vi "Constants.vi"() -> ()   [LabVIEW 2015, in "DMM-SWITCH-ScanList Shared.lvlib"]
doc: "Use this Global VI to access the GUIDs assigned to the page resources of the Custom Device."
uses:
  DMM-SWITCH-ScanList Shared.lvlib
  <instrlib>/niDMM/nidmm.llb/niDMM Function.ctl
  <instrlib>/niDMM/nidmm.llb/niDMM Resolution in Digits.ctl
  <instrlib>/niSwitch/niSwitch.LLB/niSwitch Topologies.ctl
  <instrlib>/niSwitch/niSwitch.LLB/niSwitch Trigger Input.ctl
  <instrlib>/niSwitch/niSwitch.LLB/niSwitch Scan Advanced Output.ctl
  <instrlib>/niDMM/nidmm.llb/niDMM Measurement Complete.ctl
  <instrlib>/niDMM/nidmm.llb/niDMM Trigger.ctl
panel:
  in  "Tab Control":T1(tab)
  in  "GUID Runtime Iteration":string="5260A2FF-FA1A-4B8D-AACD-153CF615834C"
  in  "GUID Runtime Error Status":string="5260A2FF-FA1A-4B8D-AACD-153CF615834C"
  in  "GUID Runtime Error Code":string="5260A2FF-FA1A-4B8D-AACD-153CF615834C"
  in  "GUID Initialization Error Status":string="5260A2FF-FA1A-4B8D-AACD-153CF615834C"
  in  "GUID Initialization Error Code":string="5260A2FF-FA1A-4B8D-AACD-153CF615834C"
  in  "GUID Scan Trigger":string="5260A2FF-FA1A-4B8D-AACD-153CF615834C"
  in  "GUID Group Ch - Runtime Status":string="813CC596-1D51-426F-B292-57396C68DA7F"
  in  "GUID Group Ch - Measurement Channels":string="3C436B89-AF05-4727-AB74-6F367A82FA29"
  in  "GUID Group Ch - Input Channels":string="247BA5C3-EBA8-4DAA-B4FA-14FAA185E47F"
  in  "GUID Group Ch - Configuration":string="5260A2FF-FA1A-4B8D-AACD-153CF615834C"
  in  "GUID Triggers Configuration Channel":string="5260A2FF-FA1A-4B8D-AACD-153CF615834C"
  in  "GUID Switch Configuration Channel":string="2CD8A1A5-3D89-4F04-ABA6-DE3C84A9E458"
  in  "GUID DMM Configuration Channel":string="F70F49EF-EA01-4EE0-9516-062BB723C6FA"
  in  "GUID DMM-SWITCH-ScanList":string="b44fa48e-2c45-4166-a547-1c211cfe843f"
  in  "Top Files Relative Path Location":string="National Instruments\\NI-DAQ\\Switch\\TopFiles"
  in  "Output Measurements Channels Path":string="Targets/Controller/Custom Devices/DMM-SWITCH-ScanList/Measurement Channels"
  in  "DMM Range Index":u16
  in  "TRIG DMM Trigger Source":string="TRIG DMM Trigger Source"
  in  "TRIG DMM Measurement Complete":string="TRIG DMM Measurement Complete"
  in  "TRIG SWITCH Scan Advanced Output":string="TRIG SWITCH Scan Advanced Output"
  in  "TRIG SWITCH Trigger Source":string="TRIG SWITCH Trigger Source"
  in  "SWITCH ListBox Channel Items":string="SWITCH ListBox Channel Items"
  in  "SWITCH ListBox Selectable Channel Items":string="SWITCH ListBox Selectable Channel Items"
  in  "SWITCH ab0":string="SWITCH ab0"
  in  "SWITCH Scan List String Mode":string="SWITCH Scan List String Mode"
  in  "SWITCH Model":string="SWITCH Model"
  in  "SWITCH Scan List":string="SWITCH Scan List"
  in  "SWITCH Generated Scan List":string="SWITCH Generated Scan List"
  in  "SWITCH Manual Scan List":string="SWITCH Manual Scan List"
  in  "SWITCH Topology":string="SWITCH Topology"
  in  "SWITCH Resource Name":string="SWITCH Resource Name"
  in  "DMM Range [EU]":string="DMM Range [EU]"
  in  "DMM Resolution in Digits":string="DMM Resolution in Digits"
  in  "DMM Measurement Type":string="DMM Measurement Type"
  in  "DMM Resource Name":string="DMM Resource Name"
  in  "SWITCH ListBox Channel Items Value":string[](array[string])
  in  "SWITCH ListBox Selectable Channel Items Value":string[](array[string])
  in  "SWITCH ab0 Value":bool
  in  "SWITCH Scan List String Mode Value":bool
  in  "SWITCH Switch Model Value":string="2503"
  in  "SWITCH Scan List Value":string
  in  "SWITCH Generated Scan List Value":string
  in  "SWITCH Manual Scan List Value":string="ab0->com0 & com0->ch0:2;"
  in  "SWITCH Topology Value":T2="2503/2-Wire 24x1 Mux" caption="SWITCH Topology"
  in  "DMM Resource Name Value":string="DMM"
  in  "SWITCH Resource Name Value":string="SWITCH"
  in  "DMM Range [EU] Value":dbl=10000.0
  in  "DMM Resolution in Digits Value":T3=6.5 caption="Resolution in Digits" items=["3 1/2"=3.5, "4 1/2"=4.5, "5 1/2"=5.5, "6 1/2"=6.5, "7 1/2"=7.5]
  in  "DMM Measurement Type Value":T4=enum."2-wire Resistance" caption="DMM Measurement Type"
  in  "TRIG SWITCH Trigger Source Value":T5=enum."TTL1" caption="TRIG Switch Trigger Source"
  in  "TRIG SWITCH Scan Advanced Output Value":T6=enum."TTL2" caption="TRIG Scan Advanced Output"
  in  "TRIG DMM Measurement Complete  Value":T7=enum."TTL 1" caption="TRIG DMM Measurement \nComplete Destination"
  in  "TRIG DMM Trigger Source Value":T8=enum."TTL 2" caption="TRIG DMM Trigger Source"
  in  "Group Ch - Runtime Status":string
  in  "Group Ch - Measurement Channels":string
  in  "Group Ch - Input Channels":string
  in  "Group Ch - Configuration":string
  in  "Runtime Status Ch - Runtime Iteration":string
  in  "Runtime Status Ch - Runtime Error Code":string
  in  "Runtime Status Ch - Runtime Error Status":string
  in  "Runtime Status Ch - Initialization Error Code":string
  in  "Runtime Status Ch - Initialization Error Status":string
  in  "Input Ch - Scan Trigger":string
  in  "Config Ch - Triggers Configuration":string
  in  "Config Ch - Switch Configuration":string
  in  "Config Ch - DMM Configuration":string
  # "DMM"
  # "SWITCH"
  # "TIMING & TRIGGERS"
  # "OUTPUT CHANNELS"
  # "CONFIGURATION"
  # "INPUT CHANNELS"
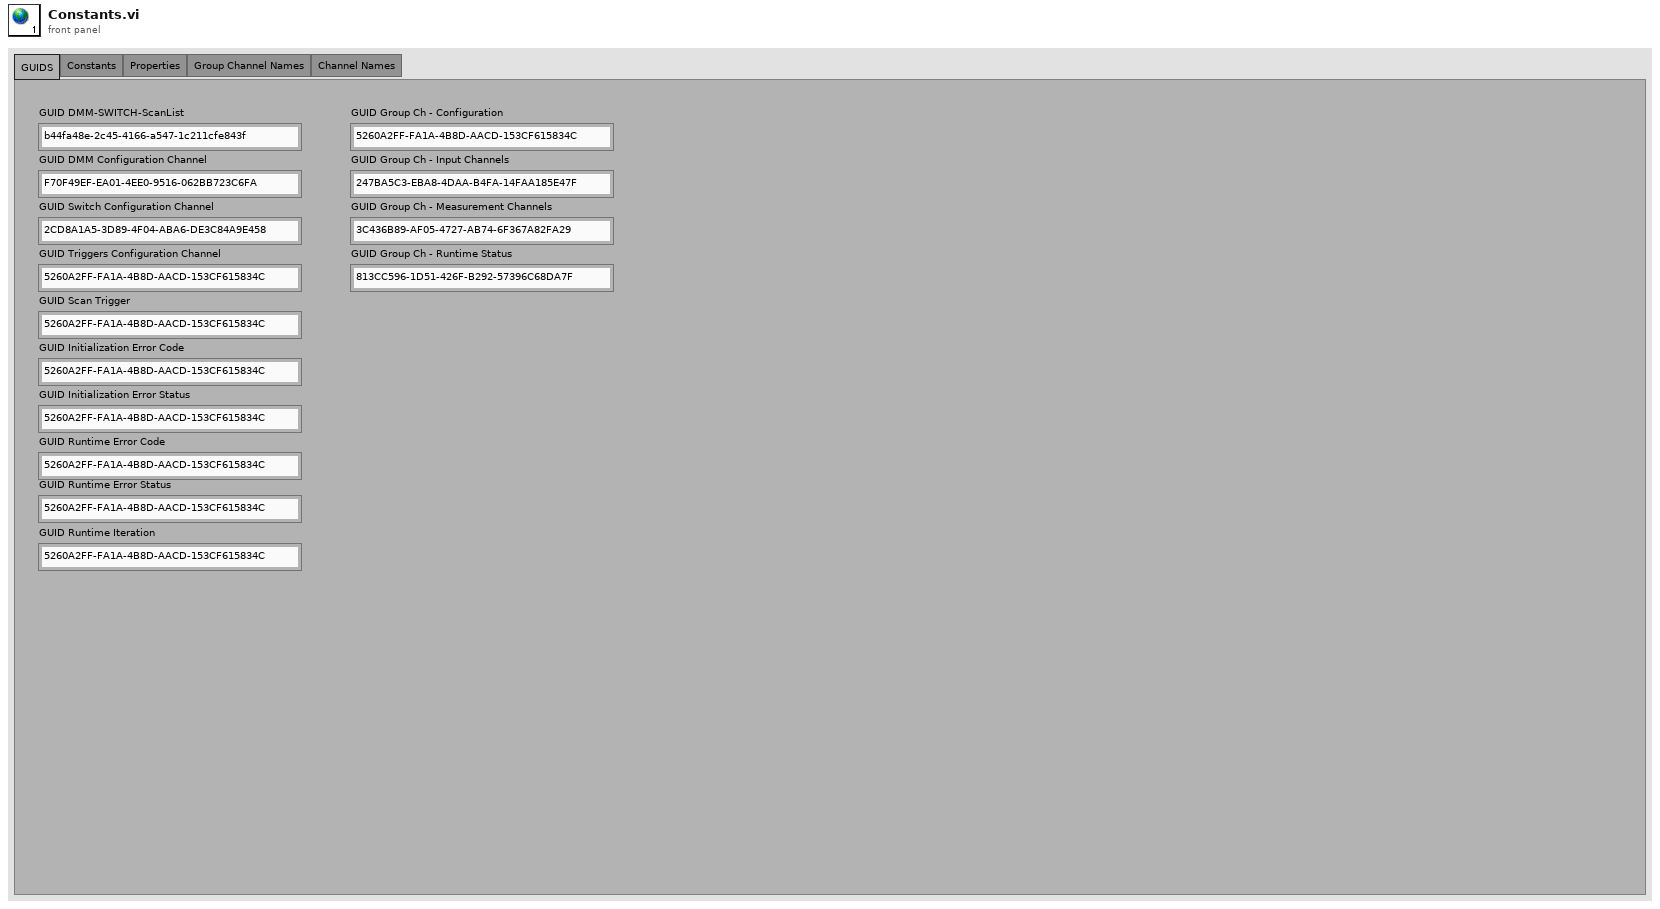
[diagram p1: front panel]
types:
  T1 = enum32{"GUIDS", "Constants", "Properties", "Group Channel Names", "Channel Names"}
  T2 = typedef "niSwitch Topologies.ctl" = string
  T3 = typedef "niDMM Resolution in Digits.ctl" = dbl
  T4 = typedef "niDMM Function.ctl" = enum16{"DC Volts", "AC Volts", "DC Current", "AC Current", "2-wire Resistance", "4-wire Resistance", "Diode", "Frequency", "Period", "AC Volts DC Coupled", "Capacitance", "Inductance", "Temperature"}
  T5 = typedef "niSwitch Trigger Input.ctl" = enum16{"Immediate", "External", "TTL0", "TTL1", "TTL2", "TTL3", "TTL4", "TTL5", "TTL6", "TTL7", "ECL0", "ECL1", "PXI Star", "Software Trigger Function", "Rear Connector", "Front Connector", "Rear Connector of Module 1", "Rear Connector of Module 2", "Rear Connector of Module 3", "Rear Connector of Module 4", "Rear Connector of Module 5", "Rear Connector of Module 6", "Rear Connector of Module 7", "Rear Connector of Module 8", "Rear Connector of Module 9", "Rear Connector of Module 10", "Rear Connector of Module 11", "Rear Connector of Module 12", "Front Connector of Module 1", "Front Connector of Module 2", "Front Connector of Module 3", "Front Connector of Module 4", "Front Connector of Module 5", "Front Connector of Module 6", "Front Connector of Module 7", "Front Connector of Module 8", "Front Connector of Module 9", "Front Connector of Module 10", "Front Connector of Module 11", "Front Connector of Module 12"}
  T6 = typedef "niSwitch Scan Advanced Output.ctl" = enum16{"None", "External", "TTL0", "TTL1", "TTL2", "TTL3", "TTL4", "TTL5", "TTL6", "TTL7", "ECL0", "ECL1", "PXI Star", "Rear Connector", "Front Connector", "Rear Connector Module 1", "Rear Connector Module 2", "Rear Connector Module 3", "Rear Connector Module 4", "Rear Connector Module 5", "Rear Connector Module 6", "Rear Connector Module 7", "Rear Connector Module 8", "Rear Connector Module 9", "Rear Connector Module 10", "Rear Connector Module 11", "Rear Connector Module 12", "Front Connector Module 1", "Front Connector Module 2", "Front Connector Module 3", "Front Connector Module 4", "Front Connector Module 5", "Front Connector Module 6", "Front Connector Module 7", "Front Connector Module 8", "Front Connector Module 9", "Front Connector Module 10", "Front Connector Module 11", "Front Connector Module 12"}
  T7 = typedef "niDMM Measurement Complete.ctl" = enum16{"None", "External", "TTL 0", "TTL 1", "TTL 2", "TTL 3", "TTL 4", "TTL 5", "TTL 6", "TTL 7", "LBR Trig 0"}
  T8 = typedef "niDMM Trigger.ctl" = enum16{"Immediate", "External", "TTL 0", "TTL 1", "TTL 2", "TTL 3", "TTL 4", "TTL 5", "TTL 6", "Software", "TTL 7", "PXI Star", "LBR Trig 1", "Aux Trig 1"}
diagram:
